vi "amplif.vi"() -> ()   [LabVIEW 2018]
uses:
  <vilib>/Plasmionique/MB Master/MB_Master_Serial/MB_Master_Serial.lvclass
  C:/Program Files/National Instruments/LabVIEW 2018/vi.lib/Plasmionique/MB Master/MB_Master/MB_Master.lvclass
  <vilib>/Plasmionique/MB Master/MB Master.lvlib
panel:
  out "error out":errorcluster
  out "Registers":u16[](array[numeric])
  in  "stop":bool
  in  "Serial Config":T1={"baud rate (bps)"=19200, "stop bits"=10, "parity"=0, "flow control"=0, "timeout"=1000, "retries"=1} {"stop bits" items=["1.0"=10, "1.5"=15, "2.0"=20]; "flow control" items=["None", "XON/XOFF", "RTS/CTS", "XON/XOFF & RTS/CTS", "DTR/DSR", "XON/XOFF & DTR/DSR"]; "parity" items=["None", "Odd", "Even", "Mark", "Space"]}
  in  "VISA Resource":refnum<visa-resource-name>
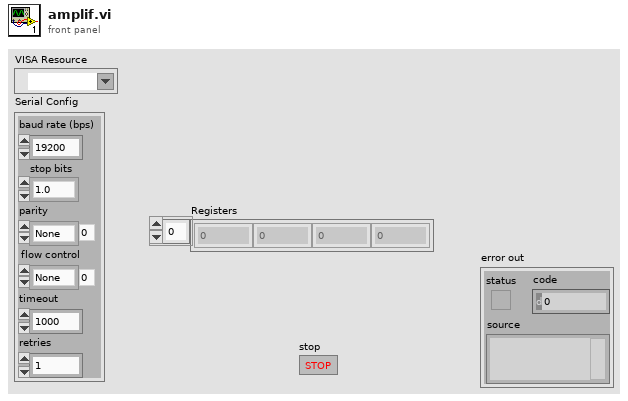
[diagram p1: front panel]
types:
  T1 = cluster{"baud rate (bps)":u32, "stop bits":u16, "parity":u16, "flow control":u16, "timeout":u32, "retries":i32}
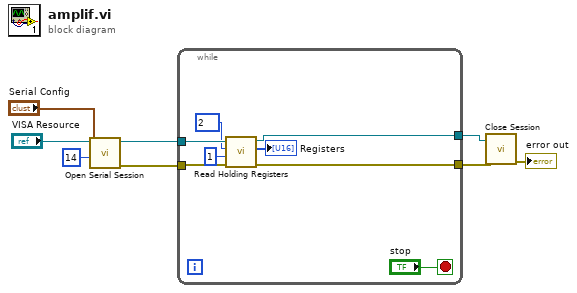
[diagram p0: block diagram]
diagram:
  n1 = call <vilib>:"Open Serial Session.vi"("Slave ID"=u8 14, "Serial Config"="Serial Config", "VISA Resource"="VISA Resource") -> ("Error out"=w4:errorcluster, "MB_Serial session"=w5:refnum<class "MB_Master_Serial.lvclass">)  [unwired: 7 in]
  n2 = while {
    tunnel: w5 -> [w15]
    tunnel: w4 -> [w14]
    tunnel: [w10] -> w3
    tunnel: [w9] -> w2
    stop <- "stop" stop-if-true
    n3 = call <vilib>:"Read Holding Registers.vi"("error in (no error)"=w14, "quantity"=u16 1, "starting address"=u16 2, "MB session in"=w15) -> ("error out"=w10:errorcluster, "Registers"=→"Registers":u16[], "MB session out"=w9:refnum<class "MB_Master_Serial.lvclass">)  [unwired: 5 in]
  }
  n4 = call-dynamic "Close Session.vi"("error in (no error)"=w3, "MB_Serial session"=w2) -> ("error out"=→"error out":errorcluster)  [unwired: 9 in]
